vi "Visual-Studio-C-Sharp-dll-Example.vi"() -> ()   [LabVIEW 2014]
uses:
  C:/Users/ASUS/Desktop/Class/MyTimerEvent/MyTimerEvent/bin/Debug/MyTimerEvent.dll
  Class/MyTimerEvent/MyTimerEvent/bin/Debug/MyTimerEvent.dll
panel:
  out "GetNumCounts":i32
  out "IntervalMs":i32
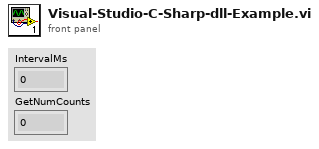
[diagram p1: front panel]
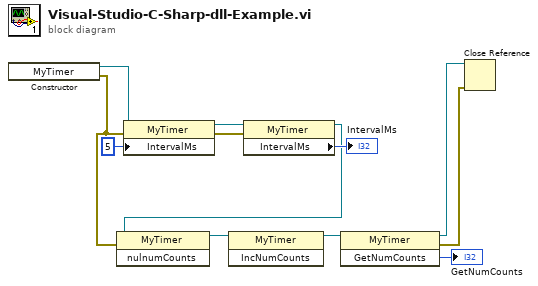
[diagram p0: block diagram]
diagram:
  n1 = constructor class="MyTimer"() -> (reference out=w12:refnum<k24>, error out=w6:errorcluster)  [unwired: 3 in, 1 out]
  n2 = property class="MyTimer"(reference=w12, error in=w6, "IntervalMs"=5) -> (reference out=w10:refnum<k24>, error out=w9:errorcluster)
  n3 = property class="MyTimer"(reference=w10, error in=w9) -> (reference out=w7:refnum<k24>, "IntervalMs"=→"IntervalMs":i32)  [unwired: 1 out]
  n4 = invoke class="MyTimer" method="nulnumCounts"(reference=w7, error in=w6) -> (reference out=w5:refnum<k24>)  [unwired: 1 in, 2 out]
  n5 = invoke class="MyTimer" method="IncNumCounts"(reference=w5) -> (reference out=w4:refnum<k24>)  [unwired: 2 in, 2 out]
  n6 = invoke class="MyTimer" method="GetNumCounts"(reference=w4) -> (reference out=w2:refnum<k24>, error out=w1:errorcluster, "GetNumCounts"=→"GetNumCounts":i32)  [unwired: 2 in]
  n7 = Close Reference(reference=w2, error in (no error)=w1) -> ()  [unwired: 1 out]
